vi "rad_Get Target Info (IP) Wrapper.vi"(6 "timeout in ms (3000)":u32=3000, 8 "error in (no error)":errorcluster, 11 "target address":string) -> (0 "error out":errorcluster, 3 "Target settings":T1={"Hostname"="", "Serial number"="", "Product name"="", "Product code"=0, "System status"="", "Credential type"=enum."None/Unlocked", "User added?"=FALSE, "Primary NIC"={"MAC address"="", "IP Address Request Mode"=2, "IP address"="", "Subnet mask"="", "Gateway"="", "DNS server"=""}} {"Primary NIC"."IP Address Request Mode" items=["Static"=1, "DHCP/Link-Local"=2, "Link-Local Only"=4, "DHCP Only"=8]})   [LabVIEW 2016]
uses:
  TypeDefs/rad_Target Information.ctl
  TypeDefs/rad_Target Network Settings.ctl
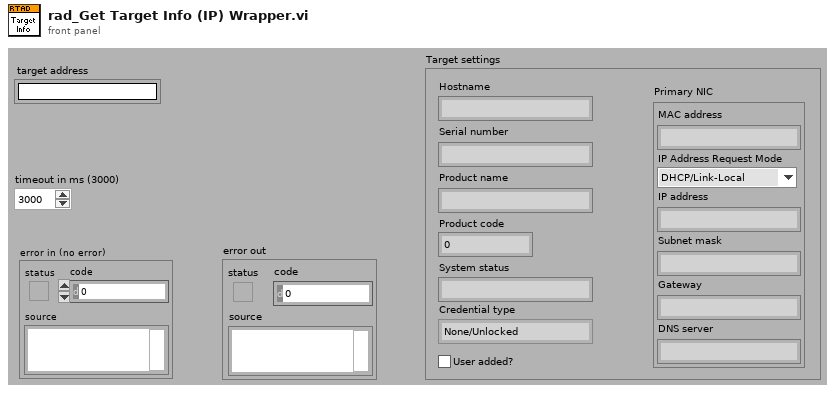
[diagram p1: front panel]
types:
  T1 = typedef "rad_Target Information.ctl" = cluster{"Hostname":string, "Serial number":string, "Product name":string, "Product code":i32, "System status":string, "Credential type":enum16{"None/Unlocked", "FTP Password", "NIAuth Credentials"}, "User added?":bool, "Primary NIC":T2}
  T2 = typedef "rad_Target Network Settings.ctl" = cluster{"MAC address":string, "IP Address Request Mode":i32, "IP address":string, "Subnet mask":string, "Gateway":string, "DNS server":string}
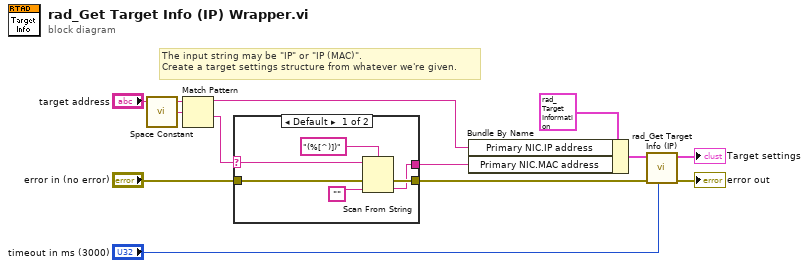
[diagram p0: block diagram]
diagram:
  # "The input string may be \"IP\" or \"IP (MAC)\".\nCreate a target settings structure from whatever we're given."
  n1 = call <vilib>:"Space Constant.vi"() -> ("String"=w9:string)
  n2 = Match Pattern(string="target address", regular expression=w9) -> (before substring=w4:string, after substring=w8:string)  [unwired: 1 in, 2 out]
  n3 = case shown="Default" w8 {
    selector: w8 -> [w17 _]
    tunnel: "error in (no error)" -> [w16 w19]
    tunnel: [w15 w19] -> w6
    tunnel: [w13 _] -> w3
    frame Default {
      n4 = Scan From String(format string="(%[^)])", input string=w17, error in=w16, default 1="") -> (error out=w15:errorcluster, output 1=w13:string)  [unwired: 1 in, 2 out]
    }
    frame "" {
    }
  }
  n5 = Bundle By Name(cluster=T1 {"Hostname"="", "Serial number"="", "Product name"="", "Product code"=0, "System status"="", "Credential type"=enum."None/Unlocked", "User added?"=FALSE, "Primary NIC"={"MAC address"="", "IP Address Request Mode"=0, "IP address"="", "Subnet mask"="", "Gateway"="", "DNS server"=""}} ("Target settings"), "Primary NIC.IP address"=w4, "Primary NIC.MAC address"=w3) -> (w2:T1)
  n6 = call "rad_Get Target Info (IP).vi"("timeout in ms (3000)"="timeout in ms (3000)", "error in (no error)"=w6, "Target settings in"=w2) -> ("error out"=→"error out":errorcluster, "Target settings out"=→"Target settings":T1)  [unwired: 7 in]
